vi "Function.vi"(8 "error in (no error)":errorcluster, 9 "Bool B":bool, 10 "Bool A":bool, 11 "OR in":refnum<class "OR_Bool.lvclass">) -> (0 "error out":errorcluster, 2 "Result":bool, 3 "OR out":refnum<class "OR_Bool.lvclass">)   [LabVIEW 2021, in "OR_Bool.lvclass"]
uses:
  OR_Bool.lvclass
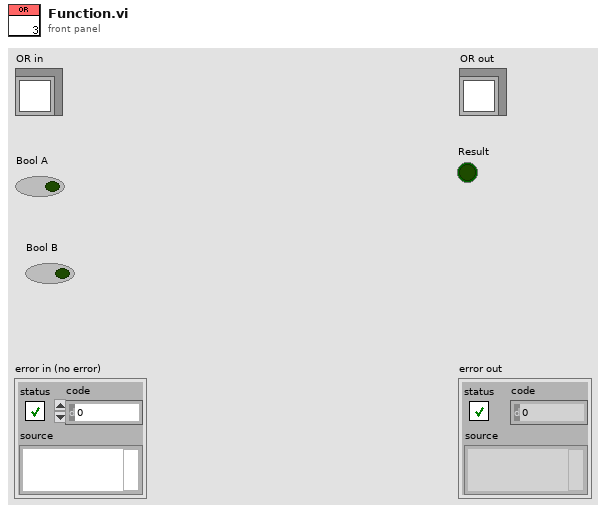
[diagram p1: front panel]
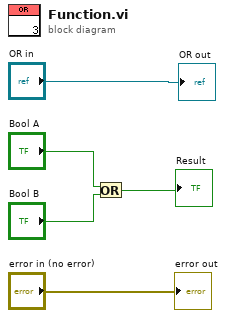
[diagram p0: block diagram]
diagram:
  n1 = Or(x="Bool A", y="Bool B") -> (x .or. y?=→"Result":bool)
  "error out" <- "error in (no error)"
  "OR out" <- "OR in"
